vi "ReadIsHomed.vi"(7 "check these axes homed":T1[](array[typedef]), 8 "error in (no error)":errorcluster, 9 "Motion Config":bool=TRUE, 11 "MotionComm in":refnum<class "MotionComm.lvclass">) -> (0 "error out":errorcluster, 1 "True = Homed":bool, 3 "MotionComm out":refnum<class "MotionComm.lvclass">)   [LabVIEW 2018, in "MotionComm.lvclass"]
uses:
  MotionComm.lvclass
  APARMainSubvis/VXM Public API/mmWaveAxis.ctl
  MotionComm.lvclass/MotionComm.ctl
  Support/MessageQue/MessageQue.lvlib
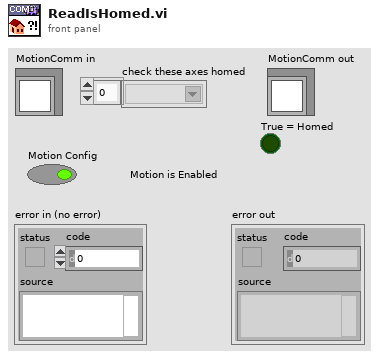
[diagram p1: front panel]
types:
  T1 = typedef "mmWaveAxis.ctl" = string
  T2 = typedef "MessageQue.lvlib/MessageQue.ctl" = refnum<queue>
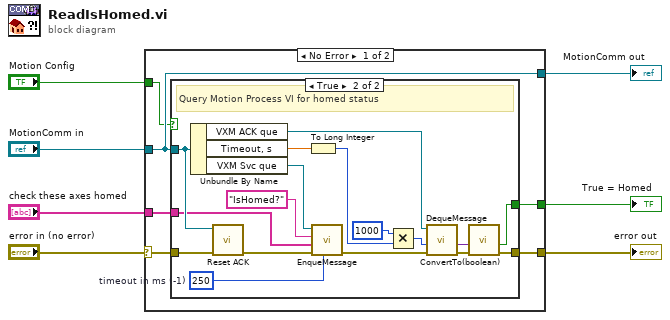
[diagram p0: block diagram]
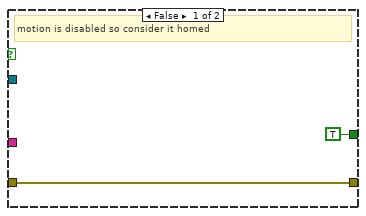
[diagram p2: hidden frame]
diagram:
  n1 = case shown="No Error" "error in (no error)" {
    selector: "error in (no error)" -> [w11 w34]
    tunnel: [w10 w34] -> w6
    tunnel: [w13 w33] -> w4
    tunnel: "MotionComm in" -> [w13 w33]
    tunnel: [w12 _] -> w3
    tunnel: "Motion Config" -> [w9 _]
    tunnel: "check these axes homed" -> [w8 _]
    frame No Error {
      n2 = case shown="True" w9 {
        tunnel: w13 -> [_ w27]
        tunnel: [TRUE ("Message Payload boolean") w25] -> w12
        tunnel: w11 -> [w15 w24]
        tunnel: [w15 w23] -> w10
        tunnel: w8 -> [_ w17]
        frame False {
          # "motion is disabled so consider it homed"
        }
        frame True {
          w16 = 250  # timeout in ms (-1)
          # "Query Motion Process VI for homed status"
          n3 = Unbundle By Name(w27) -> ("VXM ACK que"=w28:T2, "Timeout, s"=w29:dbl, "VXM Svc que"=w21:T2)
          n4 = call "Reset ACK.vi"("error in (no error)"=w24, "MotionComm in"=w27) -> ("error out"=w20:errorcluster)  [unwired: 8 in, 1 out]
          n5 = To Long Integer(number=w29) -> (32bit integer=w31:i32)
          n6 = call "EnqueMessage.vi"("timeout in ms (-1)"=w16, "error in"=w20, "Message Payload"=w17, "Message Command"="IsHomed?", "Message que"=w21) -> ("error out"=w19:errorcluster)  [unwired: 5 in, 1 out]
          n7 = Multiply(x=1000 ("timeout in ms (-1)"), y=w31) -> (x*y=w30:i32)
          n8 = call "DequeMessage.vi"("error in"=w19, "timeout in ms (-1)"=w30, "Message que"=w28) -> ("error out"=w22:errorcluster, "Message Payload"=w26:variant)  [unwired: 3 in, 4 out]
          n9 = call "ConvertTo(boolean).vi"("error in"=w22, "Message Payload"=w26) -> ("error out"=w23:errorcluster, "Message Payload boolean"=w25:bool)  [unwired: 8 in]
        }
      }
    }
    frame Error {
    }
  }
  "error out" <- w6
  "MotionComm out" <- w4
  "True = Homed" <- w3
